vi "Correction Collect.vi"(8 "error in (no error)":errorcluster, 10 "Collect Action (0: Ref)":u32(slide) max=4 step=1, 11 "VISA resource name":refnum<visa-resource-name>) -> (0 "error out":errorcluster, 3 "VISA resource name out":refnum<visa-resource-name>)   [LabVIEW 2015, in "Agilent 428X Series.lvlib"]
doc: "This function execute the cable correction data measurement to adopt the HP 4285A to individual HP 16048A/D Test Leads and calculates cable correction coefficient from the 0 m reference.\n\nNote: Model 4285 only."
uses:
  Agilent 428X Series.lvlib
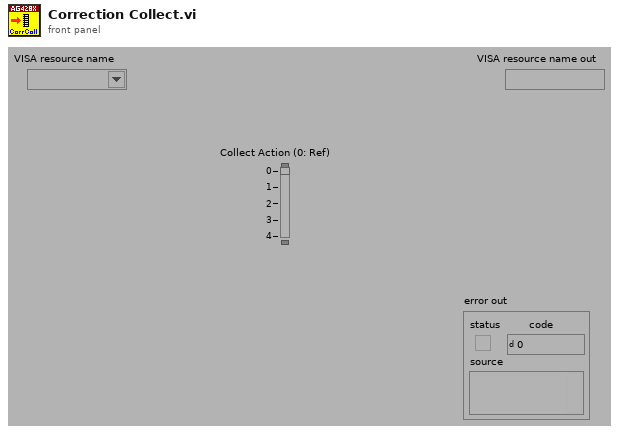
[diagram p1: front panel]
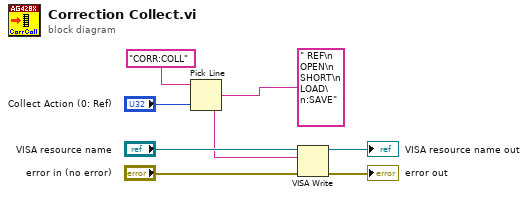
[diagram p0: block diagram]
diagram:
  n1 = Pick Line(string ("")="CORR:COLL", multi-line string=" REF\n OPEN\n SHORT\n LOAD\n:SAVE", line index="Collect Action (0: Ref)") -> (output string=w1:string)
  n2 = VISA Write(VISA resource name="VISA resource name", write buffer=w1, error in (no error)="error in (no error)") -> (VISA resource name out=→"VISA resource name out":refnum<visa-resource-name>, error out=→"error out":errorcluster)  [unwired: 1 out]
